vi "RESTful Get VI Terminal Info.vi"(5 "RESTful VI configuration":T2={"Service VI Type"=enum."Web Method", "Load VI at statup"=TRUE, "Keep VI in memory"=TRUE, "Output type"=enum."Terminal", "Output format"=enum."XML", "Use headers"=TRUE, "Buffered"=TRUE, "eng_Load VI by name"=FALSE}, 7 "context":refnum<vi>, 8 "error in":errorcluster, 11 "vi path":path) -> (0 "error out":errorcluster, 1 "Terminal Info Summary":T6[](array[typedef]), 2 "Terminal Names":string[](array[string]), 4 "Controls for XML":T1[](array[typedef]), 6 "Indicators for XML":T1[](array[typedef]))   [LabVIEW 2020]
uses:
  <vilib>/Utility/VariantDataType/VariantType.lvlib
  <vilib>/AppBuilder/Engine/RESTful INI Generator/RESTful VI Terminal Info Summary.ctl
  <resource>/Framework/Providers/Common/provcom_StringGlobals.vi
  <vilib>/AppBuilder/Engine/WebServiceDescription/LVDataTypes/LVDataTypes.lvlib
  <vilib>/AppBuilder/Engine/WebServiceDescription/LVDataTypes/LVType/LVType.lvclass
  <vilib>/AppBuilder/Engine/WebServiceDescription/Terminal Info.ctl
  <vilib>/AppBuilder/Engine/WebServiceDescription/Web Service Description.lvlib
  <vilib>/AppBuilder/AB_Classes/Source/RESTfulVI/Configure_RESTfulVI/AB_RESTful_OutputType.ctl
  <vilib>/AppBuilder/AB_Classes/Source/RESTfulVI/Configure_RESTfulVI/AB_RESTful_VIType.ctl
  <vilib>/AppBuilder/AB_Classes/Source/RESTfulVI/Configure_RESTfulVI/AB_RESTful_OutputFormat.ctl
  <vilib>/AppBuilder/AB_Classes/Source/RESTfulVI/Configure_RESTfulVI/AB_RESTful_Configuration.ctl
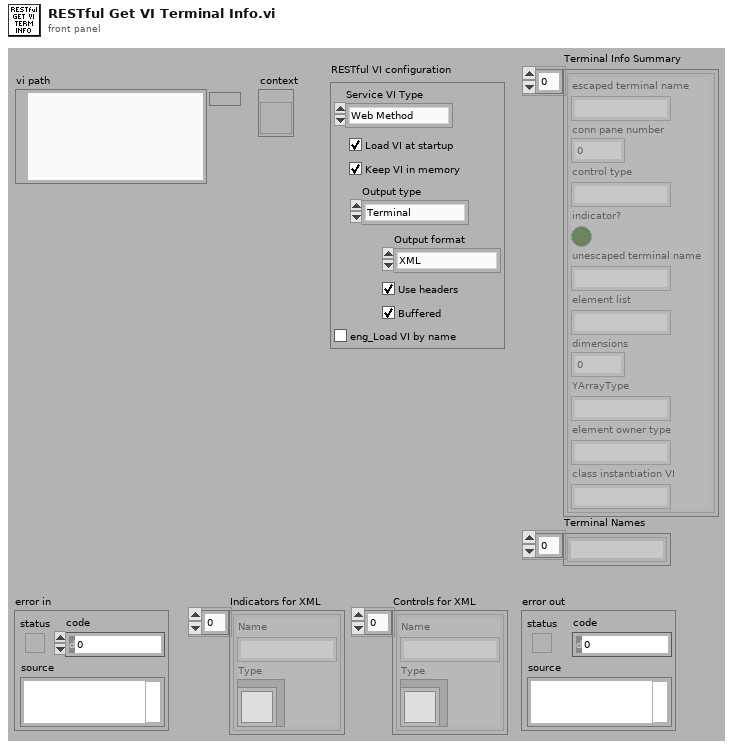
[diagram p1: front panel]
types:
  T1 = typedef "Web Service Description.lvlib/Terminal Info.ctl" = cluster{"Name":string, "Type":refnum<class "LVType.lvclass">}
  T2 = typedef "AB_RESTful_Configuration.ctl" = cluster{"Service VI Type":T3, "Load VI at statup":bool, "Keep VI in memory":bool, "Output type":T4, "Output format":T5, "Use headers":bool, "Buffered":bool, "eng_Load VI by name":bool}
  T3 = typedef "AB_RESTful_VIType.ctl" = enum32{"Web Method", "Auxiliary", "eng_Internal", "eng_Content"}
  T4 = typedef "AB_RESTful_OutputType.ctl" = enum32{"Terminal", "Stream"}
  T5 = typedef "AB_RESTful_OutputFormat.ctl" = enum32{"XML", "Text", "HTML", "JSON"}
  T6 = typedef "RESTful VI Terminal Info Summary.ctl" = cluster{"escaped terminal name":string, "conn pane number":i32, "control type":string, "indicator?":bool, "unescaped terminal name":string, "element list":string, "dimensions":u32, "YArrayType":string, "element owner type":string, "class instantiation VI":string}
  T7 = cluster{"main":string, "control ":string, "indicator":string}
  T8 = typedef "VariantType.lvlib/VIInfo.ctl" = cluster{"Data1":i16, "Data2":i16, "Flags":u32[], "Modification Date":timestamp, "Asynchronous":bool, "NonFunctional":bool, "Subroutine":bool, "SubSystem":bool}
  T9 = typedef "VariantType.lvlib/Type.ctl" = enum8{"Invalid Type", "Void", "I8", "I16", "I32", "I64", "U8", "U16", "U32", "U64", "Single Float", "Double Float", "Extended Float", "Single Complex", "Double Complex", "Extended Complex", "Enum U8", "Enum U16", "Enum U32", "Enum U64", "Single Float With Unit", "Double Float With Unit", "Extended Float With Unit", "Single Complex with Unit", "Double Complex with Unit", "Extended Complex with Unit", "Boolean", "String", "Path", "Picture", "Tag", "Array", "Cluster", "Variant", "LV Variant", "Waveform", "Timestamp", "Digital Waveform", "Digital Data", "ExpressData", "Refnum", "External Data", "VI", "Poly VI", "LabVIEW Class Instance", "Fixed Point"}
  T10 = cluster{"ArrayElt":variant, "element control name prefix":string}
  T11 = cluster{"ArrayElt":variant, "element control name prefix":string}[]
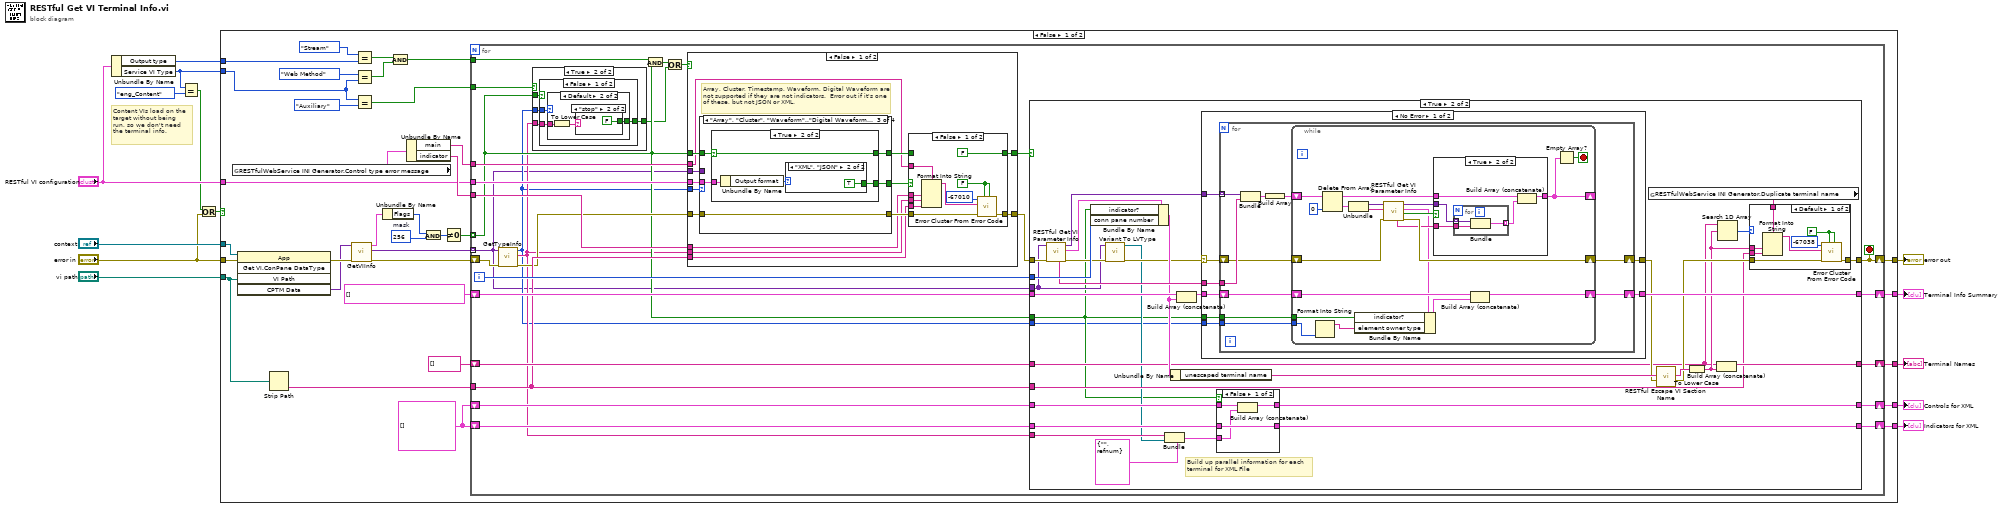
[diagram p0: block diagram]
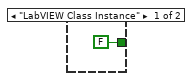
[diagram p3: hidden frame]
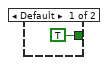
[diagram p4: hidden frame]
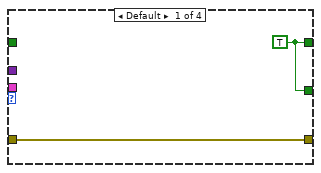
[diagram p7: hidden frame]
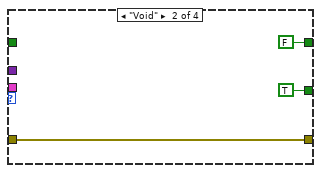
[diagram p8: hidden frame]
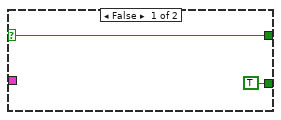
[diagram p9: hidden frame]
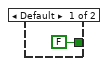
[diagram p10: hidden frame]
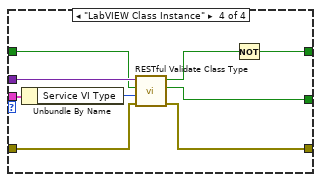
[diagram p11: hidden frame]
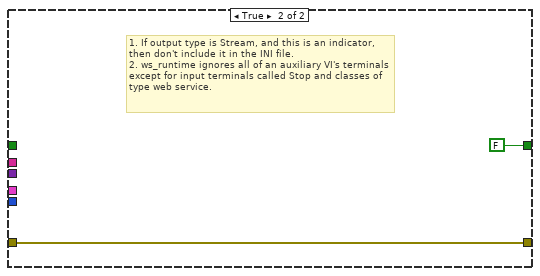
[diagram p12: hidden frame]
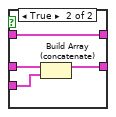
[diagram p14: hidden frame]
diagram:
  # "Content VIs load on the\ntarget without being\nrun, so we don't need\nthe terminal info."
  n1 = Unbundle By Name("RESTful VI configuration") -> ("Output type"=w4:T4, "Service VI Type"=w3:T3)
  n2 = Equal?(x=w3, y=AB_RESTful_VIType."eng_Content") -> (x = y?=w1:bool)
  n3 = Or(x=w1, y="error in") -> (x .or. y?=w7:bool)
  n4 = case shown="False" w7 {
    tunnel: [w45 _] -> w14
    tunnel: [w44 w249] -> w13
    tunnel: [w37 _] -> w12
    tunnel: "context" -> [w36 _]
    tunnel: "RESTful VI configuration" -> [w23 _]
    tunnel: "vi path" -> [w30 _]
    tunnel: [w27 _] -> w9
    tunnel: [w26 _] -> w8
    tunnel: "error in" -> [w17 w249]
    tunnel: w4 -> [w16 _]
    tunnel: w3 -> [w15 _]
    frame False {
      w28 = T1[] [] ("Outputs")
      w40 = i16 256  # mask
      n5 = global read "provcom_StringGlobals.vi" "RESTfulWebService INI Generator.Control type error message"() -> (w33:T7)
      n6 = invoke class="App" method="Get VI.ConPane DataType"(reference=w36, error in=w17, "VI Path"=w30) -> (error out=w48:errorcluster, "CPTM Data"=w47:variant)  [unwired: 2 in, 3 out]
      n7 = Strip Path(path=w30) -> (name=w29:string)  [unwired: 1 out]
      n8 = call <vilib>:"GetVIInfo.vi"("error in (no error)"=w48, "Variant"=w47) -> ("error out"=w46:errorcluster, "VI Terminal Types"=w38:variant[], "VI Info"=w42:T8)  [unwired: 7 out]
      n9 = Equal?(x=AB_RESTful_OutputType."Stream", y=w16) -> (x = y?=w22:bool)
      n10 = Equal?(x=AB_RESTful_VIType."Web Method" ("y"), y=w15) -> (x = y?=w19:bool)
      n11 = Equal?(x=w15, y=AB_RESTful_VIType."Auxiliary") -> (x = y?=w21:bool)
      n12 = Unbundle By Name(w42) -> ("Flags"=w41:u32[])
      n13 = And(x=w22, y=w19) -> (x .and. y?=w20:bool)
      n14 = Unbundle By Name(w33) -> ("main"=w32:string, "indicator"=w31:string)
      n15 = And(x=w41, y=w40) -> (x .and. y?=w43:u32[])
      n16 = Not Equal To 0?(x=w43) -> (x != 0?=w39:bool[])
      n17 = for {
        shift-right: [w74] -> w45
        shift-left: T6[] [] -> [w71]
        shift-right: [w65] -> w44
        shift-left: w46 -> [w70]
        tunnel: w39 -> [w53] mode=indexing
        tunnel: w38 -> [w49] mode=indexing
        shift-right: [w72] -> w37
        shift-left: string[] [] -> [w73]
        tunnel: w23 -> [w58]
        tunnel: w32 -> [w67]
        tunnel: w31 -> [w66]
        tunnel: w29 -> [w64]
        shift-right: [w60] -> w27
        shift-left: w28 -> [w61]
        shift-right: [w59] -> w26
        shift-left: w28 -> [w62]
        tunnel: w20 -> [w55]
        tunnel: w21 -> [w54]
        i -> [w75]
        stop <- w65 stop-if-true
        n18 = call <vilib>:"GetTypeInfo.vi"("error in (no error)"=w70, "Variant"=w49) -> ("error out"=w63:errorcluster, "Name"=w52:string, "Type Enum"=w50:T9)  [unwired: 7 out]
        n19 = case shown="True" w54 {
          tunnel: w52 -> [_ w79]
          tunnel: [_ w78] -> w51
          tunnel: w53 -> [_ w77]
          tunnel: w50 -> [_ w76]
          frame False {
          }
          frame True {
            n20 = case shown="False" w77 {
              selector: w77 -> [_ w89]
              tunnel: w79 -> [w82 _]
              tunnel: [w81 w89] -> w78
              tunnel: w76 -> [w80 _]
              frame False {
                n21 = case shown="Default" w80 {
                  tunnel: w82 -> [_ w86]
                  tunnel: [FALSE w84] -> w81
                  frame "LabVIEW Class Instance" {
                  }
                  frame Default {
                    n22 = To Lower Case(string=w86) -> (all lower case string=w85:string)
                    n23 = case shown="\"stop\"" w85 {
                      tunnel: [TRUE FALSE] -> w84
                      frame Default {
                      }
                      frame "stop" {
                      }
                    }
                  }
                }
              }
              frame True {
              }
            }
          }
        }
        n24 = And(x=w55, y=w53) -> (x .and. y?=w57:bool)
        n25 = Or(x=w57, y=w51) -> (x .or. y?=w56:bool)
        n26 = case shown="False" w56 {
          tunnel: w50 -> [w103 _]
          tunnel: [w97 FALSE] -> w69
          tunnel: [w94 w144] -> w68
          tunnel: w67 -> [w90 _]
          tunnel: w66 -> [w91 _]
          tunnel: w64 -> [w93 _]
          tunnel: w63 -> [w102 w144]
          tunnel: w52 -> [w92 _]
          tunnel: w58 -> [w101 _]
          tunnel: w53 -> [w100 _]
          tunnel: w49 -> [w99 _]
          frame False {
            # "Array, Cluster, Timestamp, Waveform, Digital Waveform are not supported if they are not indicators.  Error out if it's one of these, but not JSON or XML."
            n27 = case shown="\"Array\", \"Cluster\", \"Waveform\"..\"Digital Waveform\"" w103 {
              tunnel: w100 -> [_ _ w125 w139]
              tunnel: [w116 FALSE w123 w134] -> w98
              tunnel: w102 -> [w117 w119 w121 w141]
              tunnel: [w117 w119 w121 w140] -> w95
              tunnel: w101 -> [_ _ w124 w138]
              tunnel: w99 -> [_ _ _ w142]
              tunnel: [w116 TRUE ("valid?") w122 w136] -> w96
              frame Default {
                w116 = TRUE
              }
              frame "Void" {
              }
              frame "Array", "Cluster", "Waveform".."Digital Waveform" {
                n28 = case shown="True" w125 {
                  selector: w125 -> [w127 w129]
                  tunnel: w124 -> [_ w131]
                  tunnel: [w127 w129] -> w123
                  tunnel: [TRUE w128] -> w122
                  frame False {
                  }
                  frame True {
                    n29 = Unbundle By Name(w131) -> ("Output format"=w130:T5)
                    n30 = case shown="\"XML\", \"JSON\"" w130 {
                      tunnel: [FALSE TRUE] -> w128
                      frame Default {
                      }
                      frame "XML", "JSON" {
                      }
                    }
                  }
                }
              }
              frame "LabVIEW Class Instance" {
                n31 = Unbundle By Name(w138) -> ("Service VI Type"=w137:T3)
                n32 = call <vilib>:"RESTful Validate Class Type.vi"("error in (no error)"=w141, "Service VI Type"=w137, "indicator?"=w139, "Variant"=w142) -> ("error out"=w140:errorcluster, "valid?"=w136:bool, "ignore terminal?"=w135:bool)  [unwired: 5 in]
                n33 = Not(x=w135) -> (.not. x?=w134:bool)
              }
            }
            n34 = case shown="False" w96 {
              tunnel: w95 -> [w111 w115]
              tunnel: [w110 w115] -> w94
              tunnel: w90 -> [w108 _]
              tunnel: w91 -> [w107 _]
              tunnel: w92 -> [w106 _]
              tunnel: w93 -> [w105 _]
              tunnel: w98 -> [_ w114]
              tunnel: [FALSE w114] -> w97
              frame False {
                w113 = FALSE ("is warning? (False)")
                n35 = Format Into String(format string=w108, w107, w106, w105) -> (resulting string=w109:string)  [unwired: 2 in, 1 out]
                n36 = call <vilib>:"Error Cluster From Error Code.vi"("is warning? (False)"=w113, "show call chain? (False)"=w113, "error in (no error)"=w111, "error message (\"\")"=w109, "error code (0)"=-67010) -> ("error out"=w110:errorcluster)  [unwired: 4 out]
              }
              frame True {
              }
            }
          }
          frame True {
            # "1. If output type is Stream, and this is an indicator, then don't include it in the INI file.\n2. ws_runtime ignores all of an auxiliary VI's terminals except for input terminals called Stop and classes of type web service."
          }
        }
        n37 = case shown="True" w69 {
          tunnel: w75 -> [_ w182]
          tunnel: w53 -> [_ w153]
          tunnel: [w149 w181] -> w74
          tunnel: w73 -> [w148 w164]
          tunnel: [w148 w180] -> w72
          tunnel: w71 -> [w149 w175]
          tunnel: [w147 w166] -> w65
          tunnel: w49 -> [_ w160]
          tunnel: w68 -> [w147 w172]
          tunnel: w64 -> [_ w163]
          tunnel: w62 -> [w145 w158]
          tunnel: w61 -> [w146 w159]
          tunnel: [w146 w152] -> w60
          tunnel: [w145 w151] -> w59
          tunnel: w52 -> [_ w156]
          tunnel: w50 -> [_ w150]
          frame False {
          }
          frame True {
            # "Build up parallel information for each\nterminal for XML File"
            n38 = call <vilib>:"RESTful Get VI Parameter Info.vi"("error in (no error)"=w172, "Variant"=w160) -> ("error out"=w162:errorcluster, "Terminal Info Summary"=w179:T6, "Elements"=w178:variant[], "element control name prefix"=w177:string)  [unwired: 1 in, 5 out]
            n39 = Bundle By Name(cluster=w179, "indicator?"=w153, "conn pane number"=w182) -> (w173:T6)
            n40 = call <vilib>:"Variant To LVType.vi"("error in (no error)"=w162, "Variant"=w160) -> ("error out"=w161:errorcluster, "LVType"=w155:refnum<class "LVType.lvclass">)  [unwired: 8 out]
            n41 = Bundle(cluster=T1 {"Name"="", "Type"=refnum} ("Terminal Info"), "Name"=w156, "Type"=w155) -> (w154:T1)
            n42 = Unbundle By Name(w173) -> ("unescaped terminal name"=w176:string)
            n43 = Build Array (concatenate)(w175, w173) -> (w174:T6[])
            n44 = case shown="No Error" w161 {
              selector: w161 -> [w202 w247]
              tunnel: w178 -> [w207 _]
              tunnel: w174 -> [w204 w248]
              tunnel: w177 -> [w206 _]
              tunnel: [w205 w247] -> w168
              tunnel: [w203 w248] -> w181
              tunnel: w153 -> [w201 _]
              tunnel: w150 -> [w200 _]
              frame No Error {
                n45 = for {
                  tunnel: w207 -> [w217] mode=indexing
                  tunnel: w206 -> [w216]
                  shift-right: [w214] -> w205
                  shift-left: w202 -> [w215]
                  shift-right: [w212] -> w203
                  shift-left: w204 -> [w213]
                  tunnel: w201 -> [w209]
                  tunnel: w200 -> [w208]
                  n46 = Bundle("ArrayElt"=w217, "element control name prefix"=w216) -> (w211:T10)  [unwired: 1 out]
                  n47 = Build Array(w211) -> (w210:T11)
                  n48 = while {
                    shift-right: [w234] -> w214
                    shift-left: w215 -> [w237]
                    shift-right: [w232] -> w212
                    shift-left: w213 -> [w233]
                    shift-right: [w224] -> _
                    shift-left: w210 -> [w227]
                    tunnel: w209 -> [w220]
                    tunnel: w208 -> [w219]
                    stop <- w225 stop-if-true
                    n49 = Format Into String(w219) -> (resulting string=w218:string)  [unwired: 3 in, 1 out]
                    n50 = Delete From Array(array=w227, index=0) -> (deleted portion=w231:T10, array with subset deleted=w226:T11)  [unwired: 1 in]
                    n51 = Unbundle(w231) -> ("ArrayElt"=w230:variant, "element control name prefix"=w228:string)
                    n52 = call <vilib>:"RESTful Get VI Parameter Info.vi"("error in (no error)"=w237, "control name prefix"=w228, "Variant"=w230) -> ("error out"=w234:errorcluster, "has sub elements?"=w236:bool, "Terminal Info Summary"=w222:T6, "Elements"=w235:variant[], "element control name prefix"=w229:string)  [unwired: 4 out]
                    n53 = Bundle By Name(cluster=w222, "indicator?"=w220, "element owner type"=w218) -> (w221:T6)
                    n54 = case shown="True" w236 {
                      tunnel: w235 -> [_ w242]
                      tunnel: w226 -> [w238 w241]
                      tunnel: [w238 w240] -> w224
                      tunnel: w229 -> [_ w243]
                      frame False {
                      }
                      frame True {
                        n55 = for {
                          tunnel: w243 -> [w246]
                          tunnel: w242 -> [w245] mode=indexing
                          tunnel: [w244] -> w239 mode=indexing
                          n56 = Bundle("ArrayElt"=w245, "element control name prefix"=w246) -> (w244:T10)  [unwired: 1 out]
                        }
                        n57 = Build Array (concatenate)(w241, w239) -> (w240:T11)
                      }
                    }
                    n58 = Build Array (concatenate)(w233, w221) -> (w232:T6[])
                    n59 = Empty Array?(array=w224) -> (empty?=w225:bool)
                  }
                }
              }
              frame Error {
              }
            }
            n60 = case shown="False" w153 {
              tunnel: w159 -> [w185 w190]
              tunnel: w158 -> [w186 w189]
              tunnel: w154 -> [w183 w187]
              tunnel: [w184 w190] -> w152
              tunnel: [w186 w188] -> w151
              frame False {
                n61 = Build Array (concatenate)(w185, w183) -> (w184:T1[])
              }
              frame True {
                n62 = Build Array (concatenate)(w189, w187) -> (w188:T1[])
              }
            }
            n63 = global read "provcom_StringGlobals.vi" "RESTfulWebService INI Generator.Duplicate terminal name"() -> (w169:string)
            n64 = call <vilib>:"RESTful Escape VI Section Name.vi"("error in"=w168, "Label.Text"=w176) -> ("error out"=w167:errorcluster, "result string"=w171:string)  [unwired: 8 out]
            n65 = To Lower Case(string=w171) -> (all lower case string=w165:string)
            n66 = Build Array (concatenate)(w164, w165) -> (w180:string[])
            n67 = Search 1D Array(1D array=w164, element=w165) -> (index of element=w170:i32)  [unwired: 1 in]
            n68 = case shown="Default" w170 {
              tunnel: w167 -> [w196 w199]
              tunnel: w165 -> [w192 _]
              tunnel: [w195 w199] -> w166
              tunnel: w169 -> [w194 _]
              tunnel: w163 -> [w191 _]
              frame Default {
                w197 = FALSE ("is warning? (False)")
                n69 = Format Into String(format string=w194, w192, w191) -> (resulting string=w193:string)  [unwired: 2 in, 1 out]
                n70 = call <vilib>:"Error Cluster From Error Code.vi"("is warning? (False)"=w197, "show call chain? (False)"=w197, "error in (no error)"=w196, "error message (\"\")"=w193, "error code (0)"=-67038) -> ("error out"=w195:errorcluster)  [unwired: 4 out]
              }
              frame -1 {
              }
            }
          }
        }
      }
    }
    frame True {
    }
  }
  "Terminal Info Summary" <- w14
  "error out" <- w13
  "Terminal Names" <- w12
  "Controls for XML" <- w9
  "Indicators for XML" <- w8
